vi "Read Bool.vi"(8 "error in (no error)":errorcluster, 11 "Generic Boolean Message in":refnum<class "Generic Boolean Message.lvclass">) -> (0 "error out":errorcluster, 2 "Bool":bool, 3 "Generic Boolean Message out":refnum<class "Generic Boolean Message.lvclass">)   [LabVIEW 2017, in "Controller.lvlib" / "Generic Boolean Message.lvclass"]
uses:
  Generic Boolean Message.lvclass
  Generic Boolean Message.lvclass/Generic Boolean Message.ctl
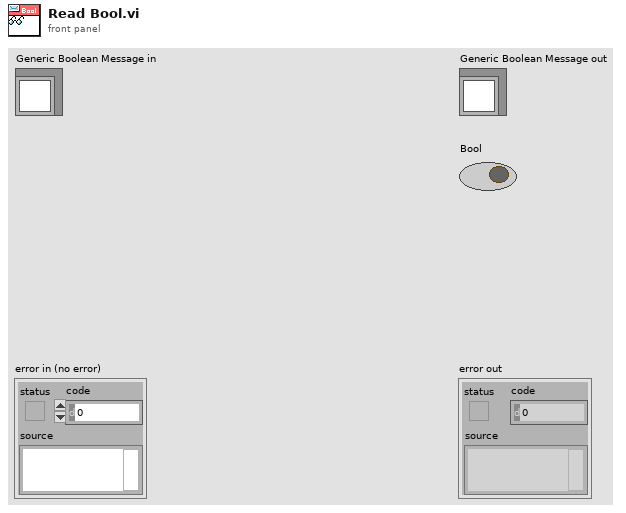
[diagram p1: front panel]
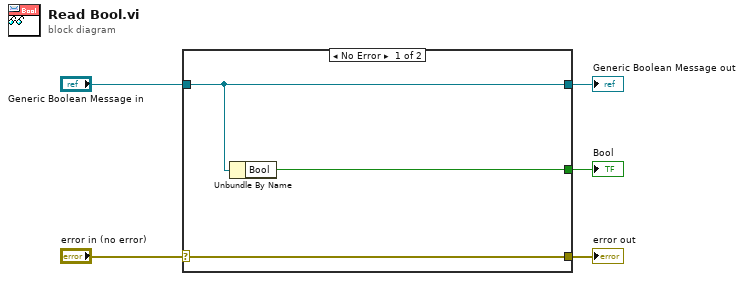
[diagram p0: block diagram]
diagram:
  n1 = case shown="No Error" "error in (no error)" {
    selector: "error in (no error)" -> [w8 w9]
    tunnel: [w8 w9] -> w4
    tunnel: [w7 w10] -> w2
    tunnel: "Generic Boolean Message in" -> [w7 w10]
    tunnel: [w6 _] -> w1
    frame No Error {
      n2 = Unbundle By Name(w7) -> ("Bool"=w6:bool)
    }
    frame Error {
    }
  }
  "error out" <- w4
  "Generic Boolean Message out" <- w2
  "Bool" <- w1
